vi "Write Log Header.vi"(8 "error in (no error)":errorcluster, 11 "Model in":refnum<class "Model.lvclass">) -> (0 "error out":errorcluster, 3 "Model out":refnum<class "Model.lvclass">)   [LabVIEW 2015, in "Model.lvclass"]
uses:
  Model.lvclass
  Model.lvclass/Model.ctl
  Test Log/Test Log/Test Log.lvclass
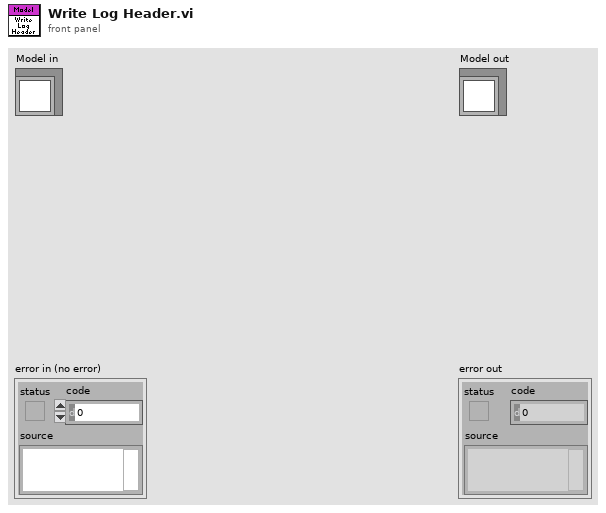
[diagram p1: front panel]
types:
  T1 = typedef "RTFAILC.lvlib/FATypes.ctl" = enum16{"SingleAxis", "LateralDualAxis", "CrossLateralDualAxis"}
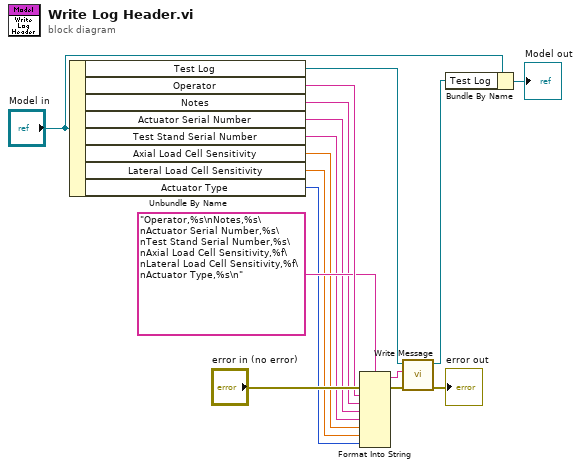
[diagram p0: block diagram]
diagram:
  n1 = Unbundle By Name("Model in") -> ("Test Log"=w15:refnum<class "Test Log.lvclass">, "Operator"=w8:string, "Notes"=w6:string, "Actuator Serial Number"=w5:string, "Test Stand Serial Number"=w4:string, "Axial Load Cell Sensitivity"=w3:dbl, "Lateral Load Cell Sensitivity"=w2:dbl, "Actuator Type"=w1:T1)
  n2 = Format Into String(format string="Operator,%s\nNotes,%s\nActuator Serial Number,%s\nTest Stand Serial Number,%s\nAxial Load Cell Sensitivity,%f\nLateral Load Cell Sensitivity,%f\nActuator Type,%s\n", error in="error in (no error)", w8, w6, w5, w4, w3, w2, w1) -> (resulting string=w16:string, error out=w12:errorcluster)  [unwired: 1 in]
  n3 = call-dynamic "Write Message.vi"("error in (no error)"=w12, "Message"=w16, "Test Log in"=w15) -> ("error out"=→"error out":errorcluster, "Test Log out"=w14:refnum<class "Test Log.lvclass">)  [unwired: 7 in]
  n4 = Bundle By Name(cluster="Model in", "Test Log"=w14) -> (→"Model out":refnum<class "Model.lvclass">)
